vi "Generate Data.vi"(8 "error in (no error)":errorcluster, 11 "Numeric Data in":refnum<class "Numeric Data.lvclass">) -> (0 "error out":errorcluster, 3 "Numeric Data out":refnum<class "Numeric Data.lvclass">)   [LabVIEW 2021, in "Numeric Data.lvclass"]
uses:
  Numeric Data.lvclass
  <vilib>/numeric/Random Number (Range) DBL.vi
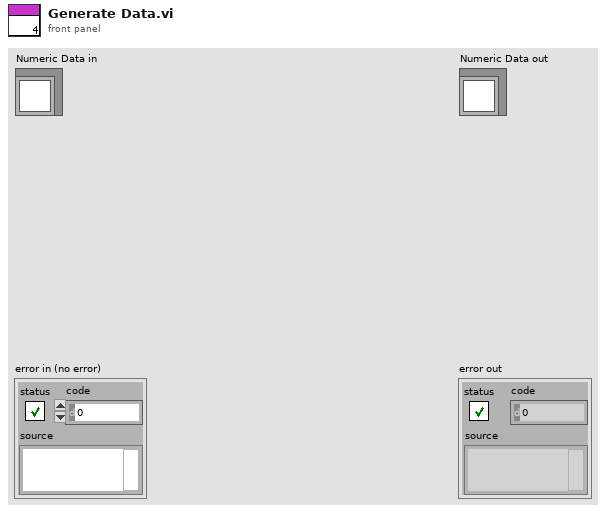
[diagram p1: front panel]
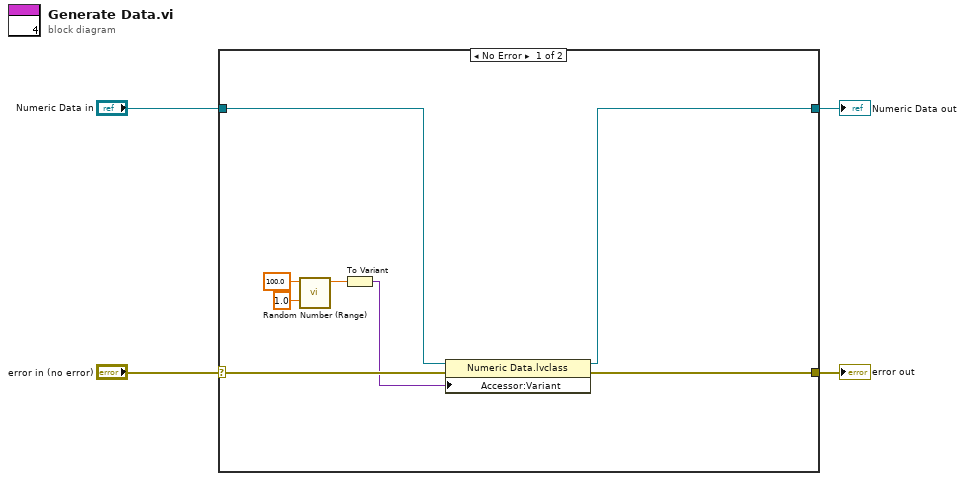
[diagram p0: block diagram]
diagram:
  n1 = case shown="No Error" "error in (no error)" {
    selector: "error in (no error)" -> [w12 w14]
    tunnel: [w8 w14] -> w3
    tunnel: [w5 w13] -> w1
    tunnel: "Numeric Data in" -> [w7 w13]
    frame No Error {
      n2 = call-poly <vilib>:"Random Number (Range).vi"("lower bound (0)"=1.0, "upper bound (100)"=100.0) -> ("number"=w9:dbl)  [unwired: 9 in]
      n3 = To Variant(anything=w9) -> (Variant=w6:variant)
      n4 = property class="Numeric Data.lvclass"(reference=w7, error in=w12, "Accessor:Variant"=w6) -> (reference out=w5:refnum<class "Numeric Data.lvclass">, error out=w8:errorcluster)
    }
    frame Error {
    }
  }
  "error out" <- w3
  "Numeric Data out" <- w1
